vi "main Interface.vi"() -> ()   [LabVIEW 2020]
uses:
  <vilib>/Simulation/Scripting/Companion Diagram/SimConfigNode/SimParams.ctl
  <vilib>/Simulation/Scripting/Companion Diagram/SimConfigNode/_simSolvers.ctl
  <vilib>/Simulation/Implementation/Shared/SIMSCR Execution Mode.ctl
  <vilib>/Simulation/Param Hierarchy/Typedefs/SIMPH Param Control Actions.ctl
  <vilib>/Simulation/Implementation/Shared/NILVSim_ParamChanged.vi
  <vilib>/Simulation/Implementation/Shared/NILVSIM_BeginStep.vi
  <vilib>/Simulation/Implementation/Shared/NILVSim_Manager.vi
  <vilib>/Utility/error.llb/Clear Errors.vi
  <vilib>/Simulation/Implementation/Shared/NILVSim_FinalizeModel.vi
  <vilib>/Simulation/Implementation/Shared/SIM Unbundle Sim Info.vi
  <vilib>/Simulation/Implementation/Shared/NILVSim_Initialize.vi
  <vilib>/Simulation/Utility/Implementation/NILVSim Get Time and IsAcceptedStep.vi
  <vilib>/Simulation/Implementation/Shared/SIMSH Read Queue.vi
  <vilib>/Simulation/Implementation/Shared/NILVSim_GetModelError.vi
  <vilib>/Simulation/Implementation/Shared/SIM Bundle Sim Info.vi
  <vilib>/Simulation/Implementation/XNodeFramework/SimXNode/SimX.xnode
  Subsystem 1.vi
  <vilib>/Simulation/Scripting/Companion Diagram/SimConfigNode/SimDog.xnode
  <vilib>/Simulation/Implementation/Shared/NI_SIM_Implementation.lvlib
panel:
  out "Time Diff":dbl[](graph)
  out "Loop Exec Time (s)":dbl
  out "Loop Wait Time (s)":dbl
  in  "stop":bool
  out "output of trf fn outside control loop y(t)":dbl
  in  "Outside sim loop input":dbl(slide) scale=0.0..10.0
  out "Transfer func 2":waveform(dbl)(graph)
  in  "Select Transfer Function Type":T1(ring)
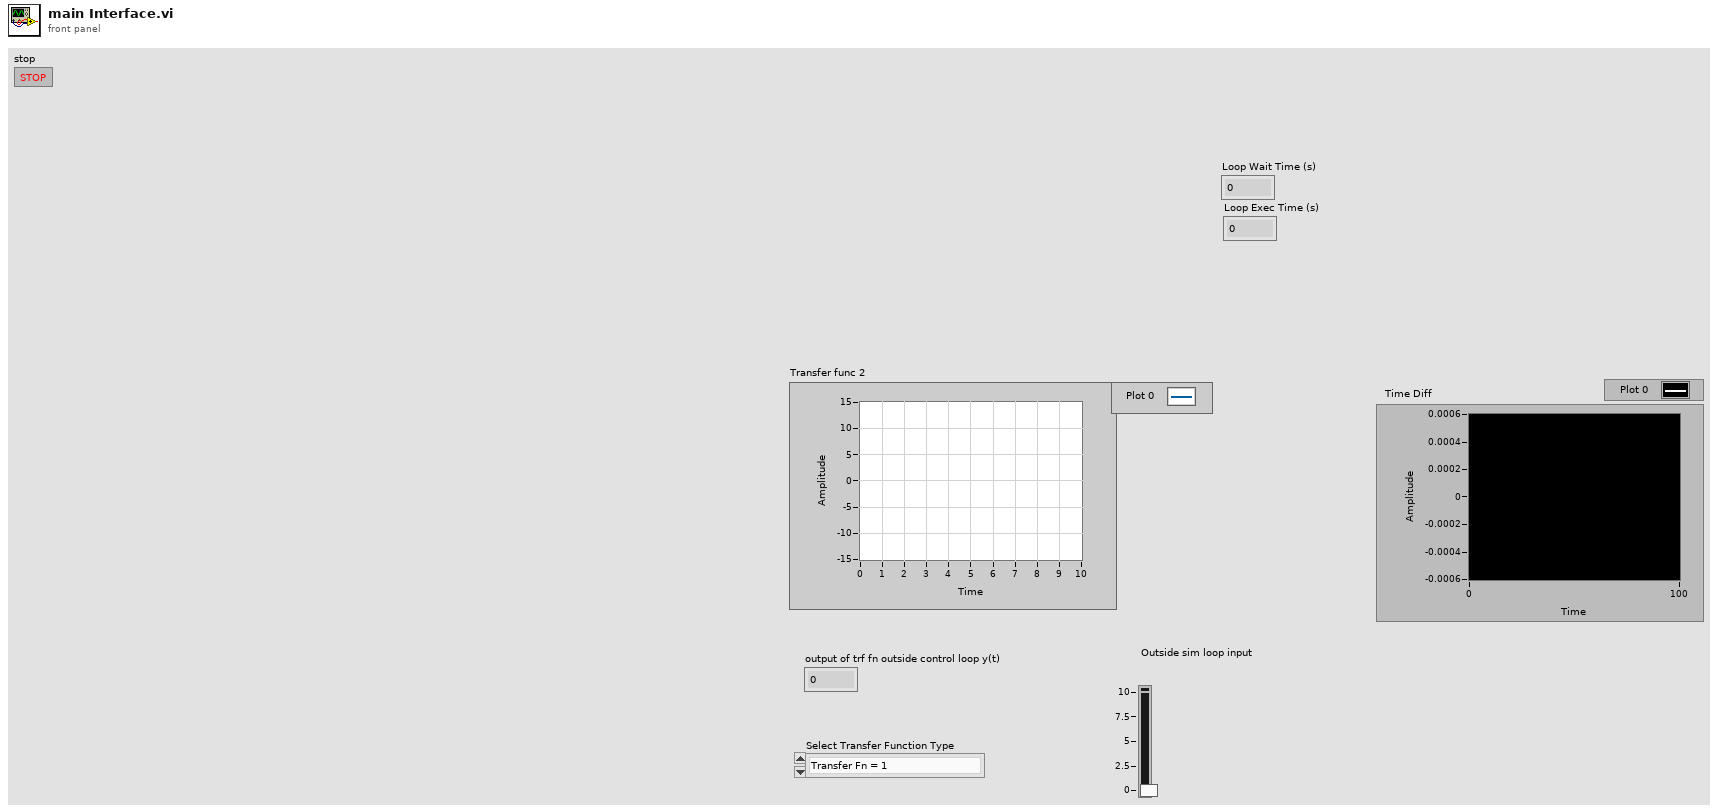
[diagram p1: front panel]
types:
  T1 = enum16{"Transfer Fn = 1", "First Order with Delay", "Second  Order Transfer Fn", "MISO Trf fn example"}
  T2 = enum16{"Simulate to Completion", "Single Time-Step Simulation (Fixed Step Only)"}
  T3 = typedef "SIMSCR Execution Mode.ctl" = enum16{"Simulate to Completion", "Single Time-Step Simulation (Fixed Step Only)"}
  T4 = typedef "SIMPH Param Control Actions.ctl" = enum16{"get params", "set params"}
  T5 = cluster{"SIMSH Sim Time":dbl, "Simulation Time Waveform":cluster{"Waveform Chart":waveform(dbl)}}
  T6 = typedef "SimParams.ctl" = cluster{"Initial Time (s)":dbl, "Final Time (s)":dbl, "Step Size (s)":dbl, "ODE Solver":T7, "Minimum Step Size (s)":dbl, "Maximum Step Size (s)":dbl, "Relative Tolerance":dbl, "Absolute Tolerance":dbl, "Software Timing":bool, "Initial Step Size (s)":dbl, "Automatic Fixed Step Size?":bool, "Automatic Discrete Step Size?":bool, "Discrete Step Size (s)":dbl, "Calculate using Time Step":bool, "Solver Wired?":bool, "Prev.Frm.Expected End":u64, "Prev.Frm.Actual End":u64, "Prev.Frm.Finished Late?":bool, "Prev.Iter.Expected End":u64, "Prev.Iter.Actual End":u64, "Prev.Iter.Finished Late?":bool, "Expected Iteration Start":u64, "Actual Iteration Start":u64, "Expected Frame Start":u64, "Actual Frame Start":u64, "Source Name":string, "Name":string, "Period":i64, "Deadline":i64, "Offset":i64, "Start":i64, "Priority":i32, "Timeout":i32, "Processor":i32, "Mode":enum32{"No Change", "Process missed periods, maintain original phase", "Discard missed periods, maintain original phase", "Process missed periods, ignore original phase", "Discard missed periods, ignore original phase"}, "Wakeup reason":enum32{"Normal", "Aborted", "Asynchronous wakeup", "Timing source error", "Timed loop error", "Timeout"}, "Error":errorcluster, "Source Type":string, "Secondary Source Type":string, "Global End Time":u64, "Global Start Time":u64, "Full Solver Reset":bool, "Execution Mode":T3, "Nan/Inf Check":bool, "Custom Solver Library":string, "Solver Is Variable":bool, "custom solver name":string, "Signal Collection Decimation":u32}
  T7 = typedef "_simSolvers.ctl" = enum16{"Runge-Kutta 1 (Euler)", "Runge-Kutta 2", "Runge-Kutta 3", "Runge-Kutta 4", "Runge-Kutta 23 (variable)", "Runge-Kutta 45 (variable)", "BDF (variable)", "Adams-Moulton (variable)", "Rosenbrock (variable)", "Discrete States Only", "SDIRK 4 (variable)", "Radau 5 (variable)", "Radau 9 (variable)", "Radau 13 (variable)", "Radau [Variable Order] (variable)", "Gear's Method (variable)", "Linearizer", "State Query", "Trim Eval", "Custom Solver"}
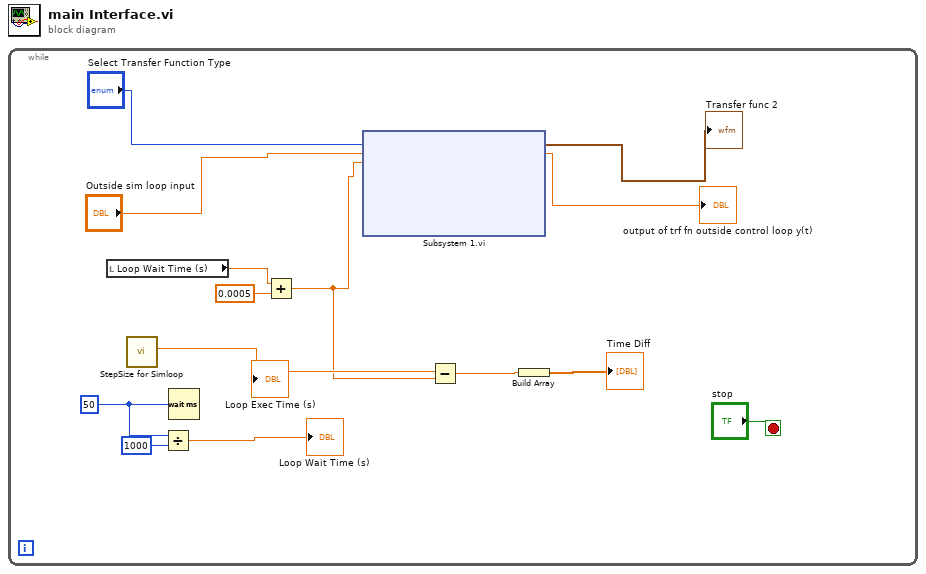
[diagram p0: block diagram]
diagram:
  n1 = while {
    stop <- "stop" stop-if-true
    w13 = u32 50 ("milliseconds to wait")
    n2 = local read "Loop Wait Time (s)"() -> (w9:dbl)
    n3 = call "StepSize for Simloop.vi"() -> ("Numeric"=w11:dbl)  [unwired: 11 in]
    "Loop Exec Time (s)" <- w11
    n4 = Divide(x=w13, y=u32 1000) -> (x/y=→"Loop Wait Time (s)":dbl)
    n5 = Wait (ms)(milliseconds to wait=w13) -> ()  [unwired: 1 out]
    n6 = Add(x=w9, y=0.0005) -> (x+y=w3:dbl)
    n7 = xnode "Subsystem 1.vi"("Select Transfer Function Type"="Select Transfer Function Type", "system input"="Outside sim loop input", "Step Size (s)"=w3) -> ("Waveform Chart"=→"Transfer func 2":waveform(dbl), "System Output"=→"output of trf fn outside control loop y(t)":dbl)  [unwired: 2 in, 9 out]
    n8 = Subtract(x=w11, y=w3) -> (x-y=w6:dbl)
    n9 = Build Array(w6) -> (→"Time Diff":dbl[])
  }
